vi "navigation parameters.vi"() -> ()   [LabVIEW 2021]
uses:
  <userlib>/Nanonis Prog Interface V5/Nanonis Prog Interface.lvlib
panel:
  in  "Turn on":bool
  in  "Turn off":bool
  in  "Coordinates":bool
  in  "Navigation":bool
  # "1.5 V\n4 kHz"
  # "1 V\n1 kHz"
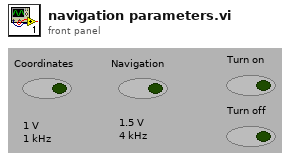
[diagram p1: front panel]
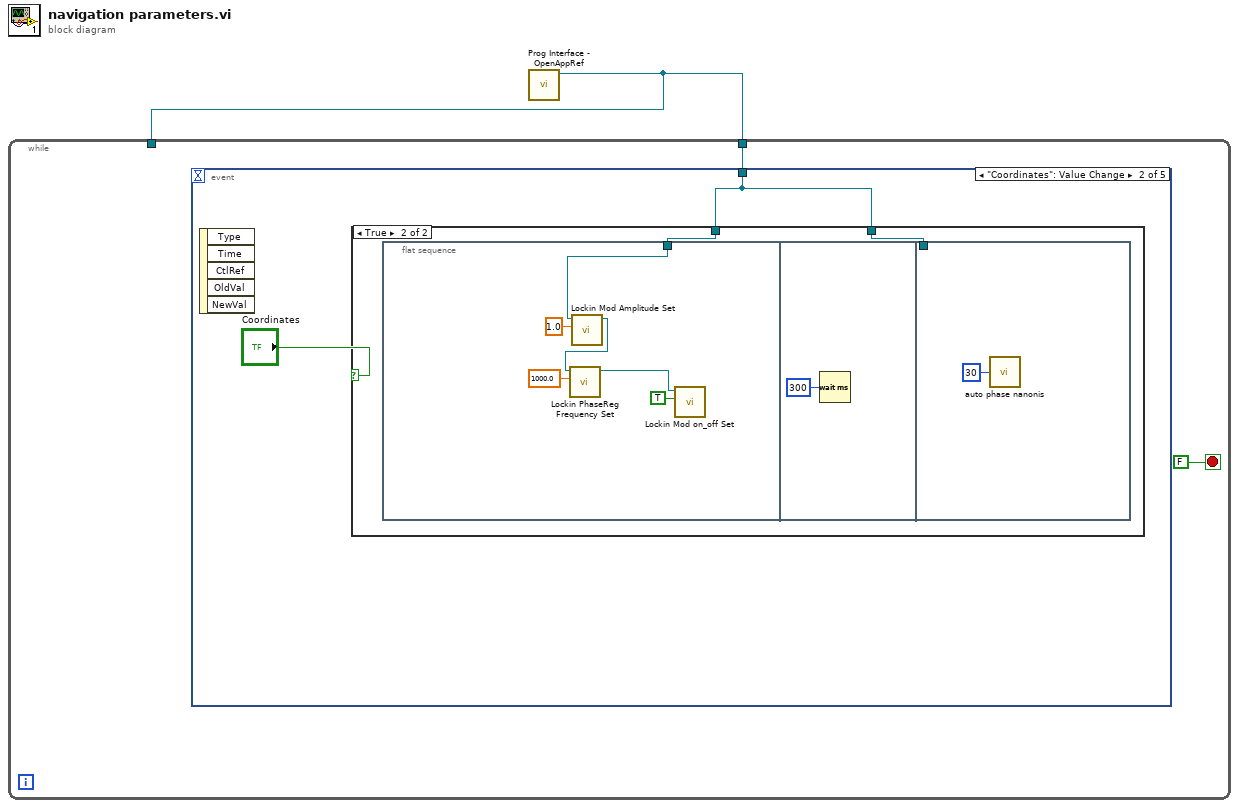
[diagram p0: block diagram]
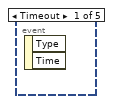
[diagram p2: hidden frame]
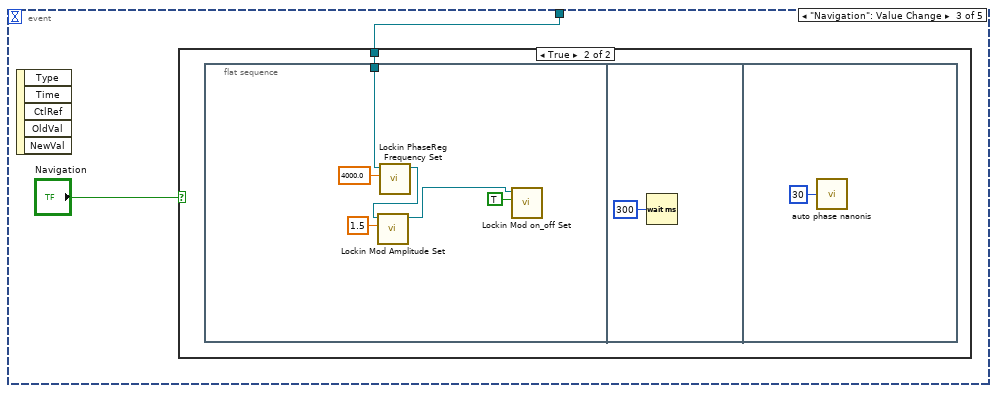
[diagram p4: hidden frame]
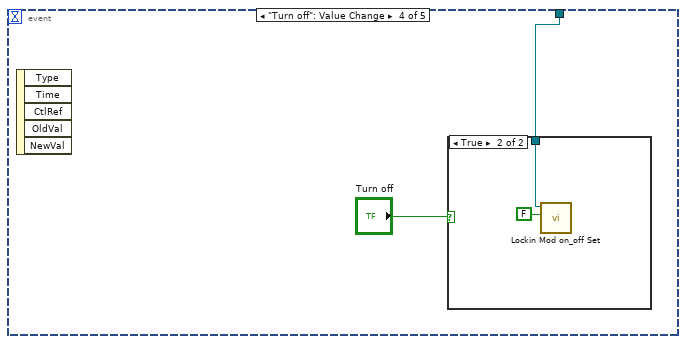
[diagram p6: hidden frame]
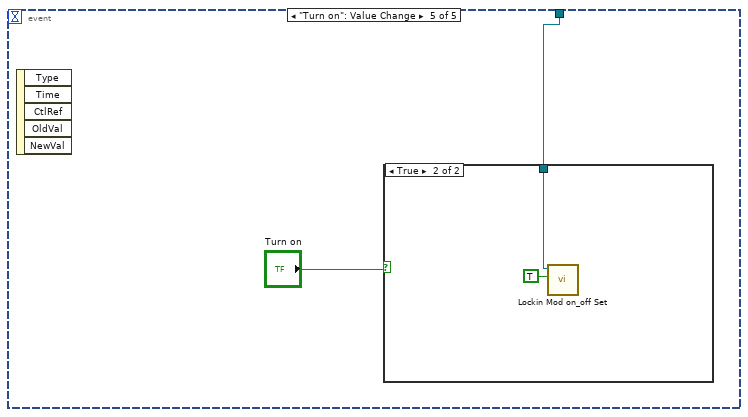
[diagram p8: hidden frame]
diagram:
  n1 = call <userlib>:"Prog Interface - OpenAppRef.vi"() -> ("Application reference"=w1:refnum<vi>)  [unwired: 6 in, 1 out]
  n2 = while {
    tunnel: w1 -> [w2]
    tunnel: w1 -> [_]
    stop <- FALSE stop-if-true
    n3 = event shown="[1] \"Coordinates\": Value Change" {
      selector: _ -> [_ _ _ _ _]
      dyn-events: _ -> [_ _ _ _ _]
      timeout: _ -> [_ _ _ _ _]
      tunnel: w2 -> [_ w4 w16 w27 w31]
      event Timeout {
        n4 = event-data() -> ()  [unwired: 1 in, 2 out]
      }
      event "Coordinates": Value Change {
        n5 = event-data() -> ()  [unwired: 1 in, 5 out]
        n6 = case shown="True" "Coordinates" {
          tunnel: w4 -> [_ w7]
          tunnel: w4 -> [_ w6]
          frame False {
          }
          frame True {
            n7 = flat-sequence {
              tunnel: w7 -> [w11]
              tunnel: w6 -> [_]
              frame #0 {
                n8 = call <userlib>:"Lockin Mod Amplitude Set.vi"("Amplitude (mod. signal unit)"=sgl 1.0, "Application ref in"=w11) -> ("Application ref out"=w10:refnum<vi>)  [unwired: 8 in, 1 out]
                n9 = call <userlib>:"Lockin PhaseReg Frequency Set.vi"("Frequency (Hz)"=1000.0, "Application ref in"=w10) -> ("Application ref out"=w8:refnum<vi>)  [unwired: 8 in, 1 out]
                n10 = call <userlib>:"Lockin Mod on_off Set.vi"("Lockin ON/OFF"=TRUE, "Application ref in"=w8) -> ()  [unwired: 8 in, 2 out]
              }
              frame #1 {
                n11 = Wait (ms)(milliseconds to wait=u32 300) -> ()  [unwired: 1 out]
              }
              frame #2 {
                n12 = call "auto phase nanonis.vi"("Num averages"=u32 30) -> ()
              }
            }
          }
        }
      }
      event "Navigation": Value Change {
        n13 = event-data() -> ()  [unwired: 1 in, 5 out]
        n14 = case shown="True" "Navigation" {
          tunnel: w16 -> [_ w18]
          frame False {
          }
          frame True {
            n15 = flat-sequence {
              tunnel: w18 -> [w19]
              frame #0 {
                n16 = call <userlib>:"Lockin PhaseReg Frequency Set.vi"("Frequency (Hz)"=4000.0, "Application ref in"=w19) -> ("Application ref out"=w22:refnum<vi>)  [unwired: 8 in, 1 out]
                n17 = call <userlib>:"Lockin Mod Amplitude Set.vi"("Amplitude (mod. signal unit)"=sgl 1.5, "Application ref in"=w22) -> ("Application ref out"=w20:refnum<vi>)  [unwired: 8 in, 1 out]
                n18 = call <userlib>:"Lockin Mod on_off Set.vi"("Lockin ON/OFF"=TRUE, "Application ref in"=w20) -> ()  [unwired: 8 in, 2 out]
              }
              frame #1 {
                n19 = Wait (ms)(milliseconds to wait=u32 300) -> ()  [unwired: 1 out]
              }
              frame #2 {
                n20 = call "auto phase nanonis.vi"("Num averages"=u32 30) -> ()
              }
            }
          }
        }
      }
      event "Turn off": Value Change {
        n21 = event-data() -> ()  [unwired: 1 in, 5 out]
        n22 = case shown="True" "Turn off" {
          tunnel: w27 -> [_ w29]
          frame False {
          }
          frame True {
            n23 = call <userlib>:"Lockin Mod on_off Set.vi"("Lockin ON/OFF"=FALSE, "Application ref in"=w29) -> ()  [unwired: 8 in, 2 out]
          }
        }
      }
      event "Turn on": Value Change {
        n24 = event-data() -> ()  [unwired: 1 in, 5 out]
        n25 = case shown="True" "Turn on" {
          tunnel: w31 -> [_ w34]
          frame False {
          }
          frame True {
            n26 = call <userlib>:"Lockin Mod on_off Set.vi"("Lockin ON/OFF"=TRUE, "Application ref in"=w34) -> ()  [unwired: 8 in, 2 out]
          }
        }
      }
    }
  }
